vi "WSVCAP SHL Host TL RFFE Stop Write Cycle.vi"(11 "error in":errorcluster) -> (15 "error out":errorcluster)   [LabVIEW 2012]
uses:
  Type Defs/WSVCAP SHL Function Enum.ctl
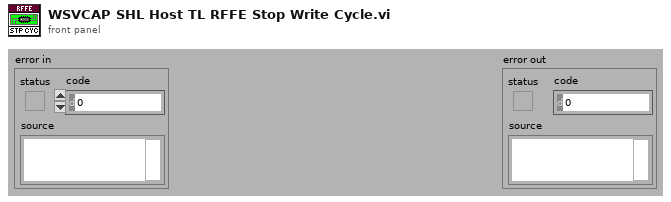
[diagram p1: front panel]
types:
  T1 = typedef "WSVCAP SHL Function Enum.ctl" = enum16{"Initialize", "Configure I2C", "Configure SPI", "Configure RFFE", "Write I2C", "Read I2C", "Write/Read SPI", "Start SPI Cycle", "Stop SPI Cycle", "Write RFFE", "Read RFFE", "Start RFFE Cycle", "Stop RFFE Cycle", "Get Status", "Close"}
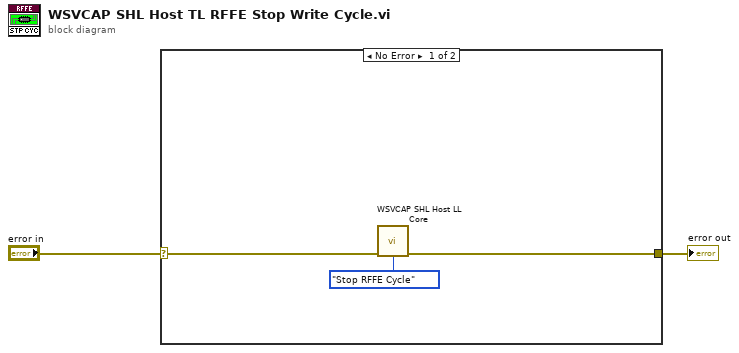
[diagram p0: block diagram]
diagram:
  n1 = case shown="No Error" "error in" {
    selector: "error in" -> [w4 _]
    tunnel: [w3 _] -> w2
    frame No Error {
      n2 = call "WSVCAP SHL Host LL Core.vi"("error in"=w4, "Function"=WSVCAP_SHL_Function_Enum."Stop RFFE Cycle") -> ("error out"=w3:errorcluster)  [unwired: 11 in, 2 out]
    }
    frame Error {
    }
  }
  "error out" <- w2
